vi "Write NHMFL Synthesizer Configuration.vi"(8 "error in (no error)":errorcluster, 10 "Configuration":T1={"DAQmx Device"="", "Variable amplitude frequency"=0.0, "Fixed amplitude frequency"=0.0, "Amplitude"=0.0, "Clock multiplier"=0, "Cannel names (variable F)"=[], "Cannel names (fixed F)"=[], "Group"="p"} {"Amplitude" format="%#_6pV"; "Fixed amplitude frequency" format="%#_6pHz"; "Variable amplitude frequency" format="%#_6pHz"}, 11 "NHMFL Synthesizer in":refnum<class "NHMFL Synthesizer.lvclass">) -> (0 "error out":errorcluster, 3 "NHMFL Synthesizer out":refnum<class "NHMFL Synthesizer.lvclass">)   [LabVIEW 2016, in "NHMFL Synthesizer.lvclass"]
uses:
  NHMFL Synthesizer.lvclass
  D:/github/Measure_core/Measure Object/Measure Object.lvclass
  NHMFL_Core/Libraries/NI-DAQ/NHMFL Synthesizer/NHMFL Synthesizer Configuration.ctl
  Measure_core/Measure Object/Measure Object.lvclass/Measure Object.ctl
  Measure_core/Measure Object/Write Configuration.vi
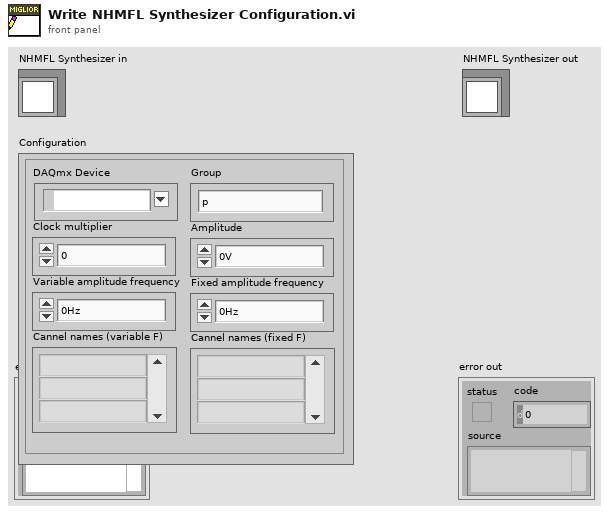
[diagram p1: front panel]
types:
  T1 = typedef "NHMFL Synthesizer Configuration.ctl" = cluster{"DAQmx Device":tag, "Variable amplitude frequency":dbl, "Fixed amplitude frequency":dbl, "Amplitude":dbl, "Clock multiplier":i32, "Cannel names (variable F)":string[], "Cannel names (fixed F)":string[], "Group":string}
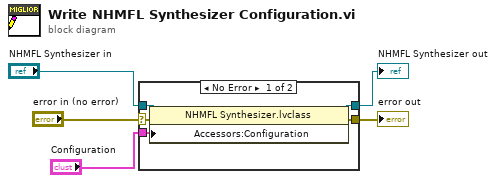
[diagram p0: block diagram]
diagram:
  n1 = case shown="No Error" "error in (no error)" {
    selector: "error in (no error)" -> [w7 w11]
    tunnel: [w6 w11] -> w4
    tunnel: [w9 w12] -> w2
    tunnel: "NHMFL Synthesizer in" -> [w10 w12]
    tunnel: "Configuration" -> [w8 _]
    frame No Error {
      n2 = property class="NHMFL Synthesizer.lvclass"(reference=w10, error in=w7, "Accessors:Configuration"=w8) -> (reference out=w9:refnum<class "NHMFL Synthesizer.lvclass">, error out=w6:errorcluster)
    }
    frame Error {
    }
  }
  "error out" <- w4
  "NHMFL Synthesizer out" <- w2
